vi "Command Editor Dialog 2.vi"(7 "Name(\"\" to use uuid)":string="Event CSM Tiny", 8 "Error in":errorcluster caption="Error in (no error)", 11 "CSM States":string="UI: Front Panel State >> Open -@ abc") -> (0 "Error out":errorcluster, 3 "Command out":string)   [LabVIEW 2017]
uses:
  user.lib/_NEVSTOP/Communicable State Machine(CSM)/_tool/_Support/def-message type.ctl
  user.lib/_NEVSTOP/Communicable State Machine(CSM)/_tool/_Support/def-Selection Type.ctl
  <vilib>/event_ctls.llb/eventvkey.ctl
  <vilib>/Utility/miscctls.llb/LVRowAndColumnUnsignedTypeDef.ctl
  user.lib/_NEVSTOP/Communicable State Machine(CSM)/AdvanceAPI/CSM - Keywords.vi
  user.lib/_NEVSTOP/Communicable State Machine(CSM)/_Support/Common/Trim Single line Text.vi
  user.lib/_NEVSTOP/Communicable State Machine(CSM)/AdvanceAPI/CSM - Break Down Multiple States String.vi
  user.lib/_NEVSTOP/Communicable State Machine(CSM)/AdvanceAPI/CSM - Compact Multiple States.vi
  user.lib/_NEVSTOP/Communicable State Machine(CSM)/Communicable State Machine.lvlib
  user.lib/_NEVSTOP/Communicable State Machine(CSM)/_tool/_Support/interfacebrowser.lvlib
  user.lib/_NEVSTOP/Communicable State Machine(CSM)/_tool/_Support/csm-tool-support.lvlib
  user.lib/_NEVSTOP/Communicable State Machine(CSM)/_csmHelper/API with lvcsm Support/CSM-Helper API with lvcsm Support.lvlib
  user.lib/_NEVSTOP/Communicable State Machine(CSM)/_csmHelper/CSM-Helper.lvclass
panel:
  out "current time":timestamp
  out "Selection":T2
  out "Msg Type":T3=enum."Message"
  in  "clear comments":bool
  in  "clear arguments":bool
  in  "->|":bool
  in  "->":bool
  in  "-@":bool
  in  "Interface-Filter":enum16{"API-Only", "UserDef States", "All"}(ring)=enum."UserDef States"
  in  "Candidates":i32(listbox)
  in  "MainTree":string(tree)
  in  "CSM-States":i32(listbox)
  in  "Comments":string
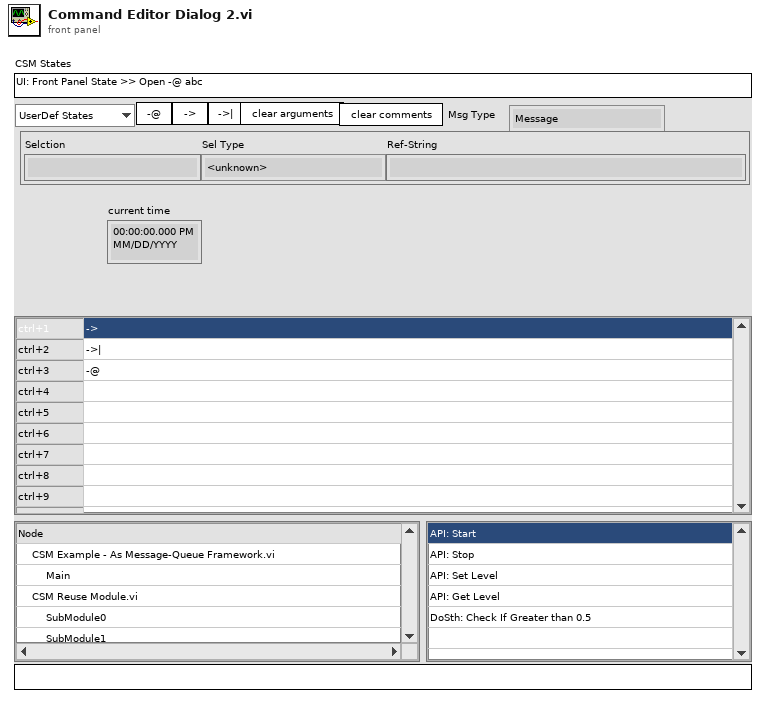
[diagram p1: front panel]
types:
  T1 = typedef "def-Selection Type.ctl" = enum16{"<unknown>", "State-StateOrSignal", "State-ArgSymbol", "State-Arg", "Reg-Oper", "Reg-Symbol", "Msg-State", "Msg-Arg", "Msg-ArgSymbol", "Msg-Symbol", "Msg-Module", "Broadcast-Signal", "Broadcast-ArgSymbol", "Broadcast-Arg", "Broadcast-Symbol", "Broadcast-Oper", "Comment-Symbol", "Comment-Content"}
  T2 = cluster{"Selction":string, "Sel Type":T1, "Ref-String":string}
  T3 = typedef "def-message type.ctl" = enum16{"State", "Message", "Broadcast", "Registration"}
  T4 = enum32{"Invalid", "Standard", "Closed", "Hidden", "Minimized", "Maximized"}
  T5 = enum32{"invalid app kind", "Development System", "Run Time System", "Student Edition", "Embedded LabVIEW", "Evaluation", "Custom"}
  T6 = typedef "LVRowAndColumnUnsignedTypeDef.ctl" = cluster{"Row":u32, "Column":u32}
  T7 = cluster{"Opton:All-CSM-VIs":bool, "Option:Online Only":bool}
  T8 = typedef "Communicable State Machine.lvlib/_CSM_Response Source Message.ctl" = cluster{"‘State":string, "’Arguments":string, "’Error":errorcluster}
  T9 = cluster{"Core":cluster{"Current VI Reference":refnum<vi>, "Close Panel on Exit?":bool}, "CSM States":string, "Selection":cluster{"end":i32, "start":i32}, "Msg Type":T3, "Selection":cluster{"Selction":string, "Sel Type":T1, "Ref-String":string}}
  T10 = typedef "LVPoint32TypeDef.ctl" = cluster{"Horizontal":i32, "Vertical":i32}
  T11 = typedef "eventvkey.ctl" = enum16{"ASCII", "Enter", "Return", "Shift", "Ctrl", "Alt", "Cmd", "Opt", "Caps", "NumLock", "Clear", "Break", "Up", "Down", "Left", "Right", "Insert", "Delete", "Home", "End", "PageUp", "PageDown", "Escape", "Help", "Pause", "ScrollLock", "F1", "F2", "F3", "F4", "F5", "F6", "F7", "F8", "F9", "F10", "F11", "F12", "F13", "F14", "F15", "F16", "F17", "F18", "F19", "F20", "F21", "F22", "F23", "F24", "Play", "VolumeUp", "VolumeDown", "Mute", "Two Byte Char"}
  T12 = cluster{"Shift":bool, "Ctrl":bool, "Alt":bool, "Cmd":bool, "Opt":bool}
  T13 = cluster{"Current VI Reference":refnum<vi>, "Close Panel on Exit?":bool}
  T14 = typedef "LVSelectionTypeDef.ctl" = cluster{"Selection Start":u32, "Selection End":u32}
  T15 = cluster{"single-line text":string, "single-line text":string}
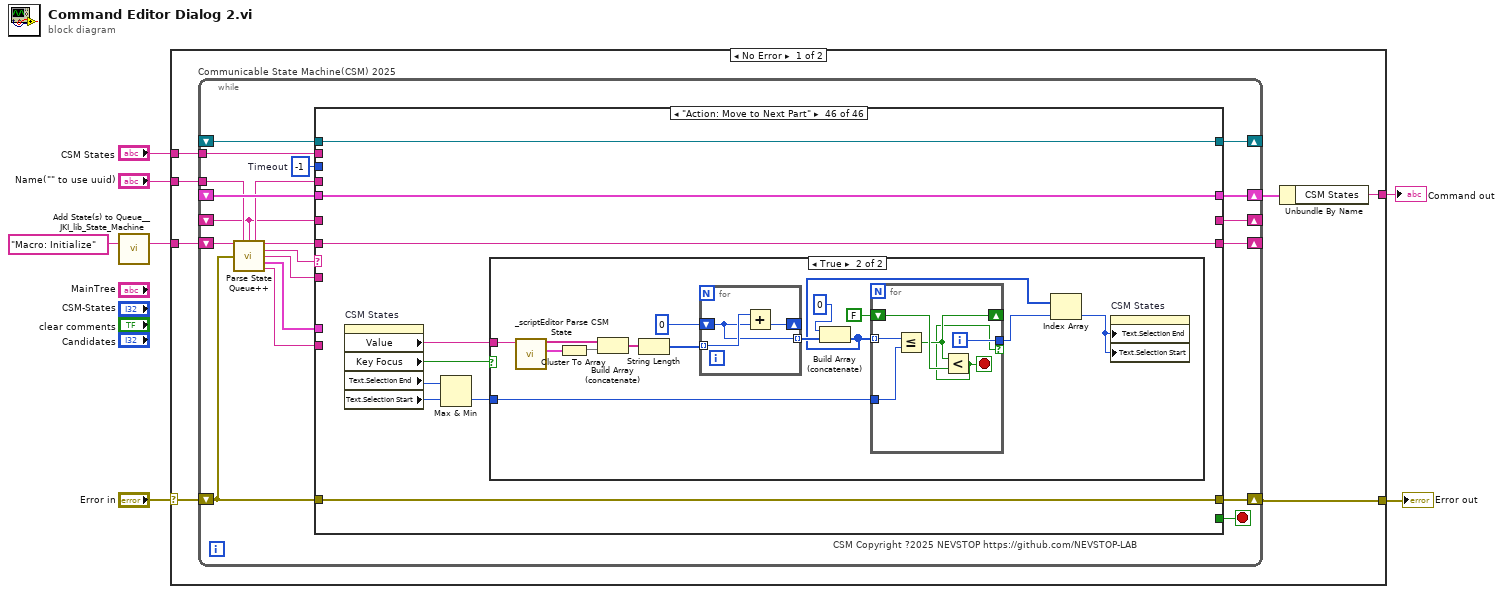
[diagram p0: block diagram]
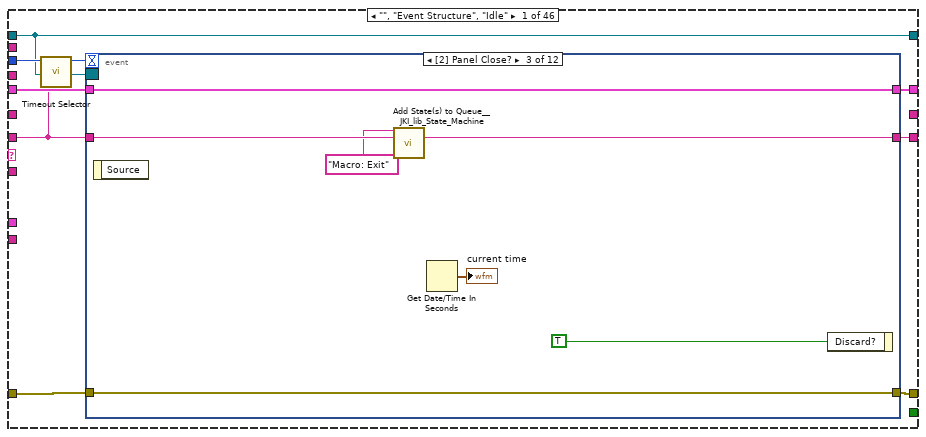
[diagram p2: hidden frame]
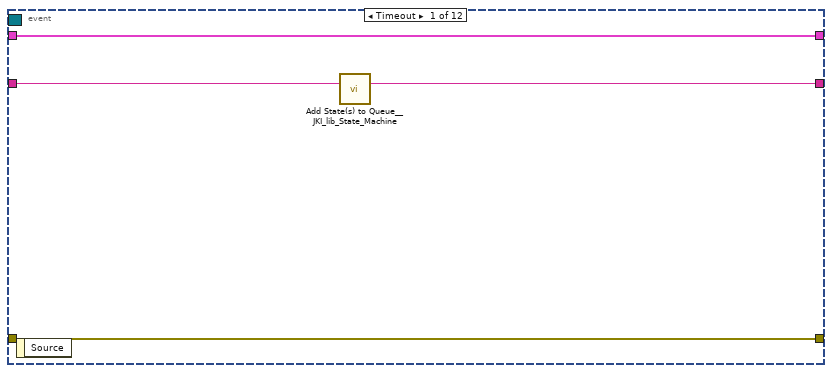
[diagram p3: hidden frame]
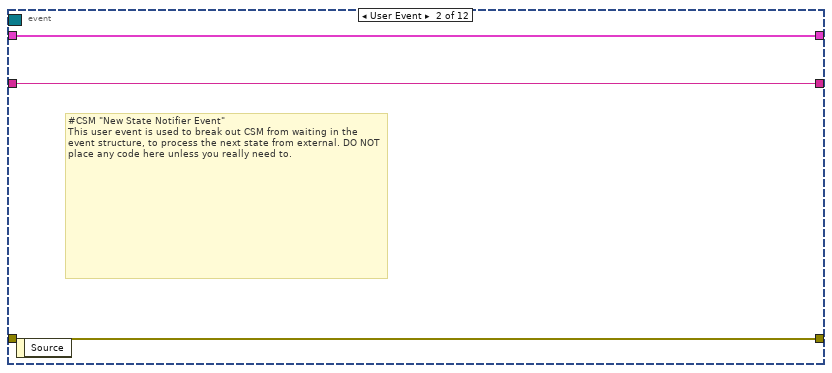
[diagram p4: hidden frame]
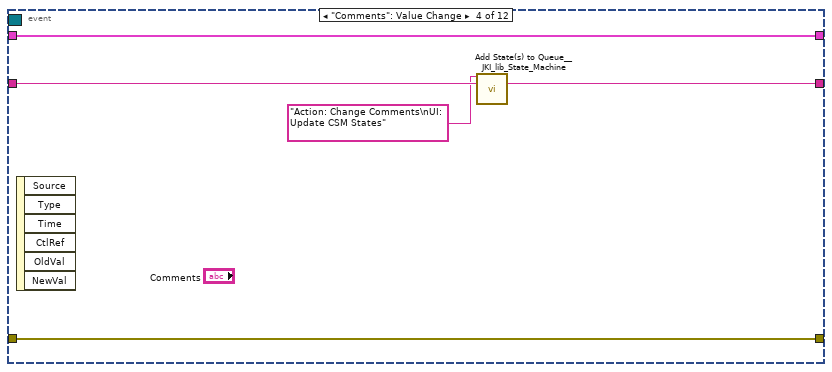
[diagram p5: hidden frame]
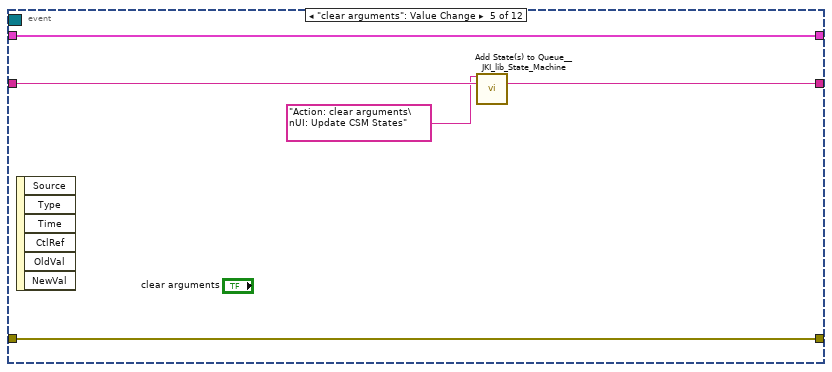
[diagram p6: hidden frame]
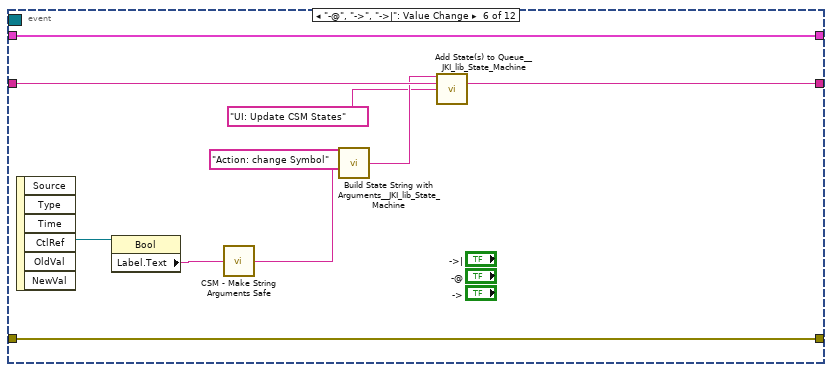
[diagram p7: hidden frame]
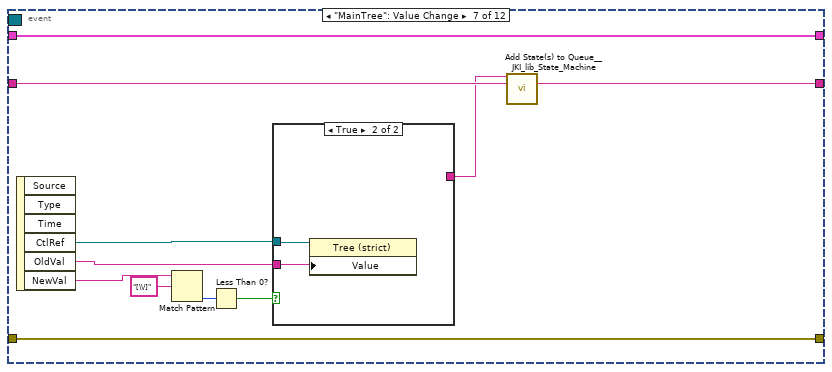
[diagram p8: hidden frame]
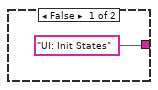
[diagram p9: hidden frame]
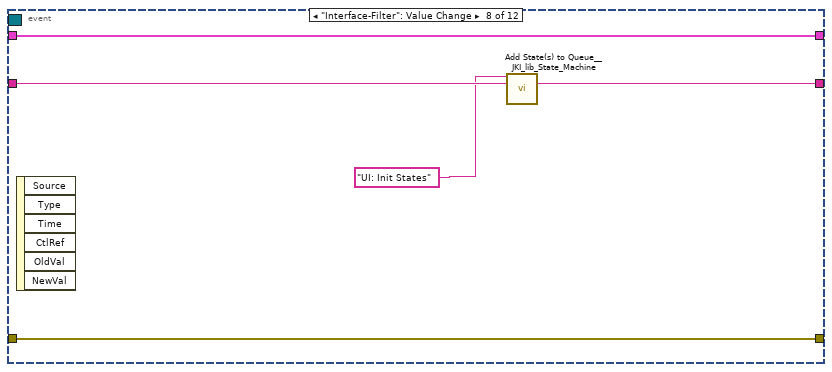
[diagram p10: hidden frame]
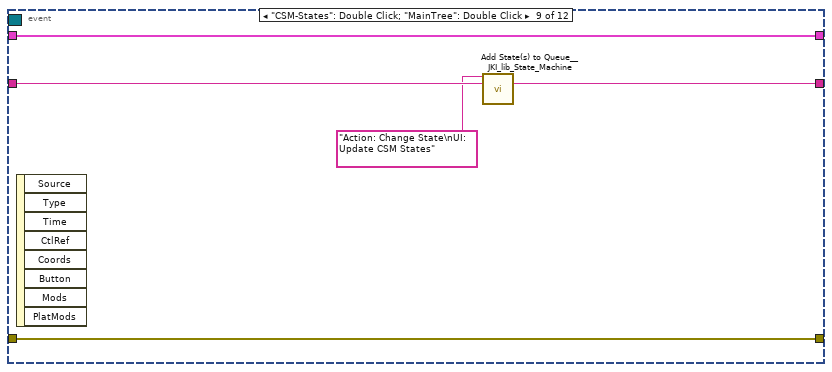
[diagram p11: hidden frame]
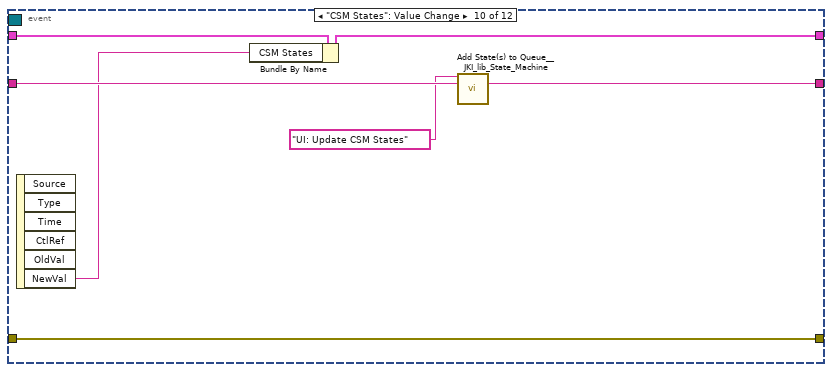
[diagram p12: hidden frame]
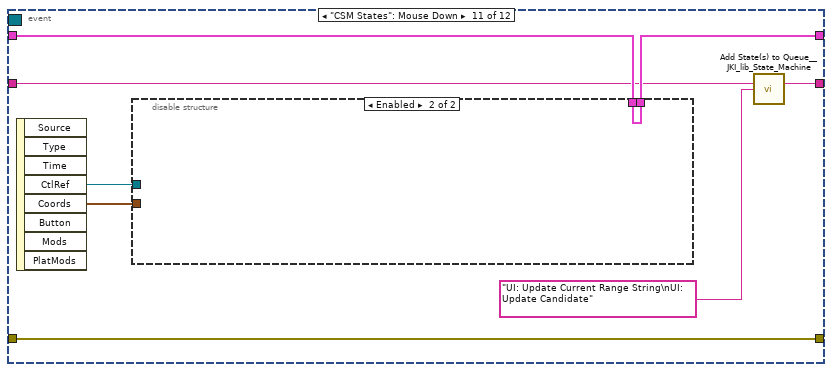
[diagram p13: hidden frame]
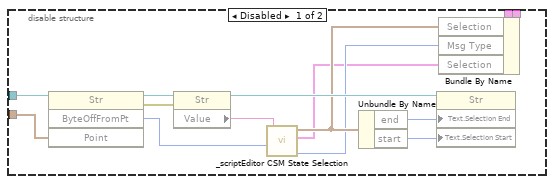
[diagram p14: hidden frame]
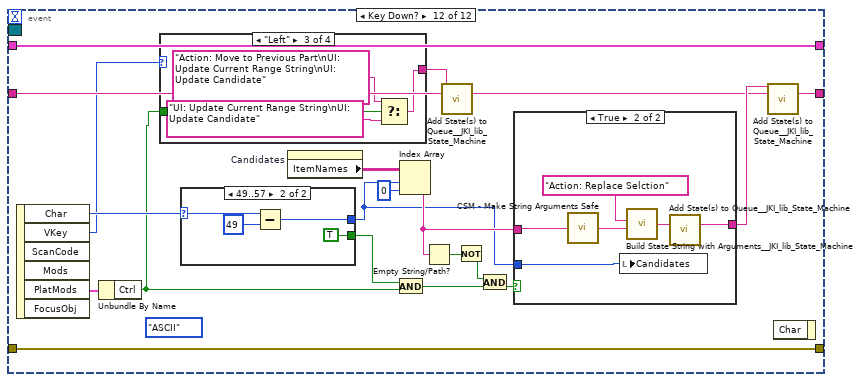
[diagram p15: hidden frame]
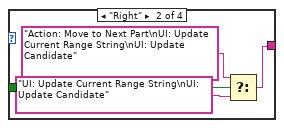
[diagram p17: hidden frame]
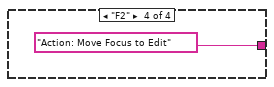
[diagram p18: hidden frame]
diagram:
  n1 = call <vilib>:"Add State(s) to Queue__JKI_lib_State_Machine.vi"("State(s) in (\"\")"="Macro: Initialize" ("Init State(\"Macro: Initialize\")")) -> ("States Out"=w7:string)  [unwired: 14 in]
  n2 = case shown="No Error" "Error in" {
    selector: "Error in" -> [w11 w791]
    tunnel: w7 -> [w14 _]
    tunnel: "Name(\"\" to use uuid)" -> [w13 _]
    tunnel: [w12 w791] -> w4
    tunnel: [w9 w790] -> w1
    tunnel: "CSM States" -> [w8 w790]
    frame No Error {
      n3 = while "Communicable State Machine(CSM) 2025" {
        shift-right: [w29] -> w10
        shift-left: _ -> [w28]
        shift-right: [w32] -> w12
        shift-left: w11 -> [w26]
        shift-right: [w31] -> _
        shift-left: w14 -> [w33]
        tunnel: w13 -> [w22]
        shift-right: [w25] -> _
        shift-left: _ -> [w16]
        shift-right: [w24] -> _
        shift-left: _ -> [w23]
        tunnel: w8 -> [w15]
        stop <- w30 stop-if-true
        w27 = -1  # Timeout
        # "CSM Copyright ?2025 NEVSTOP https://github.com/NEVSTOP-LAB"
        n4 = call "Parse State Queue++.vi"("State Queue"=w33, "Name(\"\" to use uuid)"=w22, "Response Arguments"=w16, "Previous Error"=w26) -> ("Name Used"=w17:string, "Remaining States"=w34:string, "Current State"=w21:string, "Arguments"=w20:string, ">> Response Source Message >>"=w19:T8, ">> Source CSM >>"=w18:string)  [unwired: 6 in]
        n5 = case shown="\"Action: Move to Next Part\"" w21 {
          selector: w21 -> [_ _ _ w182 _ _ _ _ _ _ _ _ _ _ _ _ _ _ _ _ _ _ _ _ _ _ _ _ _ _ _ _ _ _ _ _ _ _ _ _ _ _ _ _ _ _]
          tunnel: w34 -> [w35 w173 w179 w187 w194 w200 w223 w229 w236 w245 w258 w273 w279 w284 w294 w301 w306 w313 w317 w323 w331 w346 w367 w384 w402 w418 w491 w503 w507 w511 w523 w540 w546 w558 w561 w564 w576 w585 w605 w640 w668 w695 w700 w709 w732 w765]
          tunnel: w20 -> [_ _ _ _ _ w199 w218 w228 w235 w244 _ _ _ _ _ _ _ _ _ _ _ _ _ _ w397 w412 _ _ _ _ _ _ _ _ _ w566 _ _ w595 _ _ w688 _ _ _ _]
          tunnel: w28 -> [w42 w172 w176 w185 w193 w204 w224 w231 w238 w247 w257 w266 w277 w281 _ w296 w303 w312 w316 w320 w327 w345 w366 w387 w400 w414 w489 w497 w506 w510 w521 w537 w543 w555 w560 w570 w573 w583 w603 w638 w666 w692 w699 w708 w731 w764]
          tunnel: [w41 w174 w177 w180 w195 errorcluster {"status"=FALSE, "code"=0, "source"=""} ("error out") w219 w226 w233 w250 w259 w270 w276 w282 w291 w297 w304 w307 w315 w321 w329 w347 w368 w395 w398 w415 w492 w504 w508 w512 w524 w538 w544 w556 w562 w571 w574 w586 w606 w641 w669 w696 w701 w710 w733 w766] -> w32
          tunnel: w26 -> [w40 w174 w177 w188 w195 w201 w225 w227 w234 _ w259 w270 w276 w282 w291 w298 w304 _ w318 w321 w329 w347 w368 w395 w399 w416 w492 w504 w508 w512 w524 w538 w544 w556 w562 w571 w574 w586 w606 w641 w669 w696 w701 w710 w733 w766]
          tunnel: [w43 w173 w178 w186 w194 w196 w222 w232 w239 w246 w258 w272 w278 w283 w293 w300 w305 w313 w317 w322 w330 w346 w367 w385 w401 w417 w491 w503 w507 w511 w523 w539 w545 w557 w561 w565 w575 w585 w605 w640 w668 w695 w700 w709 w732 w765] -> w31
          tunnel: [_ _ _ _ _ _ TRUE _ _ _ _ _ TRUE _ _ _ _ _ _ _ _ _ _ _ _ _ _ _ _ _ _ _ _ _ _ _ _ _ _ _ _ _ _ _ _ _] -> w30
          tunnel: [w39 w172 w176 w185 w193 w204 w224 w231 w238 w248 w257 w271 w277 w281 w292 w296 w303 w312 w316 w320 w327 w345 w366 w387 w400 w414 w489 w496 w506 w510 w521 w537 w543 w555 w560 w568 w573 w579 w600 w635 w663 w693 w699 w708 w731 w764] -> w29
          tunnel: w27 -> [w38 _ _ _ _ _ _ _ _ _ _ _ _ _ _ _ _ _ _ _ _ _ _ _ _ _ _ _ _ _ _ _ _ _ _ _ _ _ _ _ _ _ _ _ _ _]
          tunnel: w18 -> [_ _ _ _ _ _ _ _ _ w242 _ _ _ _ _ _ _ _ _ _ _ _ _ _ _ _ _ _ _ _ _ _ _ _ _ _ _ _ _ _ _ _ _ _ _ _]
          tunnel: w19 -> [_ _ _ _ _ _ _ _ _ w249 _ _ _ _ _ _ _ _ _ _ _ _ _ _ _ _ _ _ _ _ _ _ _ _ _ _ _ _ _ _ _ _ _ _ _ _]
          tunnel: [_ _ _ "" w189 _ _ _ _ _ _ _ _ _ _ _ _ _ _ _ _ _ _ _ _ _ _ _ _ _ _ _ _ _ _ _ _ _ _ _ _ _ _ _ _ _] -> w25
          tunnel: [w37 w171 w175 w183 w192 w203 w220 w230 w237 w251 w256 w260 w274 w280 w289 w295 w302 w311 w314 w319 w328 w344 w365 w394 w396 w411 w490 w502 w505 w509 w522 w536 w541 w548 w559 w569 w572 w584 w604 w639 w667 w694 w698 w707 w730 w763] -> w24
          tunnel: w23 -> [w37 w171 w175 w183 w192 w203 w220 w230 w237 w251 w256 w260 w274 w280 w289 w295 w302 _ w314 w319 w328 w344 w365 w394 w396 w411 w490 w502 w505 w509 w522 w536 w541 w548 w559 w569 w572 w584 w604 w639 w667 w694 w698 w707 w730 w763]
          tunnel: w17 -> [_ _ _ w181 _ _ w217 _ _ _ _ _ _ _ _ _ _ w310 _ _ _ _ _ _ _ _ _ _ _ _ _ _ _ _ _ _ _ _ _ _ _ _ _ _ _ _]
          tunnel: w16 -> [_ _ _ _ _ _ _ _ _ _ _ _ _ _ _ _ _ _ _ _ _ _ _ _ _ _ _ _ _ _ _ _ _ _ _ _ _ _ _ _ _ _ _ _ _ _]
          tunnel: w15 -> [_ _ _ _ _ _ _ _ _ _ _ _ _ _ w288 _ _ _ _ _ _ _ _ _ _ _ _ _ _ _ _ _ _ _ _ _ _ _ _ _ _ _ _ _ _ _]
          frame "", "Event Structure", "Idle" {
            n6 = call "Timeout Selector.vi"("Remaining States"=w35, "Timeout Expected"=w38) -> ("Timeout"=w36:i32)  [unwired: 5 in]
            n7 = event shown="[2] Panel Close?" {
              selector: w37 -> [_ _ _ _ _ _ _ _ _ _ _ _]
              dyn-events: _ -> [_ _ _ _ _ _ _ _ _ _ _ _]
              timeout: w36 -> [_ _ _ _ _ _ _ _ _ _ _ _]
              tunnel: w35 -> [w47 w49 w57 w59 w64 w74 w79 w93 w98 w105 w110 w136]
              tunnel: [w46 w49 w56 w60 w65 w75 w80 w94 w99 w106 w111 w147] -> w43
              tunnel: w42 -> [w44 w50 w54 w61 w66 w76 w87 w95 w100 w107 w115 w150]
              tunnel: [w45 w48 w55 w62 w67 w77 w88 w96 w101 w108 w116 w151] -> w41
              tunnel: w40 -> [w45 w48 w55 w62 w67 w77 w88 w96 w101 w108 w116 w151]
              tunnel: [w44 w50 w54 w61 w66 w76 w87 w95 w100 w103 w112 w150] -> w39
              event Timeout {
                n8 = event-data() -> ()  [unwired: 1 in, 1 out]
                n9 = call <vilib>:"Add State(s) to Queue__JKI_lib_State_Machine.vi"("State(s) in (\"\")"=w47) -> ("States Out"=w46:string)  [unwired: 14 in]
              }
              event User Event {
                # "#CSM \"New State Notifier Event\"\nThis user event is used to break out CSM from waiting in the event structure, to process the next state from external. DO NOT place any code here unless you really need to."
                n10 = event-data() -> ()  [unwired: 1 in, 1 out]
              }
              event Panel Close? {
                n11 = event-data() -> ()  [unwired: 1 in, 1 out]
                n12 = call <vilib>:"Add State(s) to Queue__JKI_lib_State_Machine.vi"("State(s) in Front (\"\")"="Macro: Exit", "State(s) in (\"\")"=w57) -> ("States Out"=w56:string)  [unwired: 13 in]
                n13 = Get Date/Time In Seconds() -> (seconds since 1Jan1904=→"current time":timestamp)
                n14 = event-data("Discard?"=TRUE) -> ()  [unwired: 1 in, 1 out]
              }
              event "Comments": Value Change {
                n15 = event-data() -> ()  [unwired: 1 in, 6 out]
                n16 = call <vilib>:"Add State(s) to Queue__JKI_lib_State_Machine.vi"("State(s) in Front (\"\")"="Action: Change Comments\nUI: Update CSM States" ("State(s) in Front (\"\")"), "State(s) in (\"\")"=w59) -> ("States Out"=w60:string)  [unwired: 13 in]
              }
              event "clear arguments": Value Change {
                n17 = event-data() -> ()  [unwired: 1 in, 6 out]
                n18 = call <vilib>:"Add State(s) to Queue__JKI_lib_State_Machine.vi"("State(s) in Front (\"\")"="Action: clear arguments\nUI: Update CSM States" ("State(s) in Front (\"\")"), "State(s) in (\"\")"=w64) -> ("States Out"=w65:string)  [unwired: 13 in]
              }
              event "-@", "->", "->|": Value Change {
                n19 = event-data() -> ("CtlRef"=w71:refnum<vi>)  [unwired: 1 in, 5 out]
                n20 = property class="Bool"(reference=w71) -> ("Label.Text"=w70:string)  [unwired: 1 in, 2 out]
                n21 = call "CSM - Make String Arguments Safe.vi"("Argurment String"=w70) -> ("Safe Argurment String"=w69:string)  [unwired: 8 in]
                n22 = call <vilib>:"Build State String with Arguments__JKI_lib_State_Machine.vi"("Arguments (\"\")"=w69, "State"="Action: change Symbol") -> ("State with Arguments"=w73:string)  [unwired: 4 in]
                n23 = call <vilib>:"Add State(s) to Queue__JKI_lib_State_Machine.vi"("State(s) in Front (\"\")"=w73, "State(s) in (\"\")"=w74, "State(s) at Back (\"\")"="UI: Update CSM States" ("State")) -> ("States Out"=w75:string)  [unwired: 12 in]
              }
              event "MainTree": Value Change {
                n24 = event-data() -> ("CtlRef"=w82:refnum<vi>, "OldVal"=w81:string, "NewVal"=w86:string)  [unwired: 1 in, 3 out]
                n25 = Match Pattern(string=w86, regular expression="[\\/]") -> (offset past match=w84:i32)  [unwired: 1 in, 3 out]
                n26 = Less Than 0?(x=w84) -> (x < 0?=w83:bool)
                n27 = case shown="True" w83 {
                  tunnel: w82 -> [_ w91]
                  tunnel: w81 -> [_ w90]
                  tunnel: ["UI: Init States" ("State(s) in Front (\"\")") _] -> w78
                  frame False {
                  }
                  frame True {
                    n28 = property class="Tree (strict)"(reference=w91, "Value"=w90) -> ()  [unwired: 1 in, 2 out]
                  }
                }
                n29 = call <vilib>:"Add State(s) to Queue__JKI_lib_State_Machine.vi"("State(s) in Front (\"\")"=w78, "State(s) in (\"\")"=w79) -> ("States Out"=w80:string)  [unwired: 13 in]
              }
              event "Interface-Filter": Value Change {
                n30 = event-data() -> ()  [unwired: 1 in, 6 out]
                n31 = call <vilib>:"Add State(s) to Queue__JKI_lib_State_Machine.vi"("State(s) in Front (\"\")"="UI: Init States" ("State(s) in Front (\"\")"), "State(s) in (\"\")"=w93) -> ("States Out"=w94:string)  [unwired: 13 in]
              }
              event "CSM-States", "MainTree": Double Click {
                n32 = event-data() -> ()  [unwired: 1 in, 8 out]
                n33 = call <vilib>:"Add State(s) to Queue__JKI_lib_State_Machine.vi"("State(s) in Front (\"\")"="Action: Change State\nUI: Update CSM States" ("State(s) in Front (\"\")"), "State(s) in (\"\")"=w98) -> ("States Out"=w99:string)  [unwired: 13 in]
              }
              event "CSM States": Value Change {
                n34 = event-data() -> ("NewVal"=w102:string)  [unwired: 1 in, 5 out]
                n35 = Bundle By Name(cluster=w107, "CSM States"=w102) -> (w103:T9)
                n36 = call <vilib>:"Add State(s) to Queue__JKI_lib_State_Machine.vi"("State(s) in Front (\"\")"="UI: Update CSM States" ("State(s) in Front (\"\")"), "State(s) in (\"\")"=w105) -> ("States Out"=w106:string)  [unwired: 13 in]
              }
              event "CSM States": Mouse Down {
                n37 = event-data() -> ("CtlRef"=w114:refnum<vi>, "Coords"=w113:T10)  [unwired: 1 in, 6 out]
                n38 = disable-structure shown="Enabled" {
                  disable-tunnel: w115 -> [w130 w131]
                  disable-tunnel: w114 -> [w129 _]
                  disable-tunnel: w113 -> [w128 _]
                  disable-tunnel: [w120 w131] -> w112
                  frame Disabled {
                    n39 = invoke class="Str" method="ByteOffFromPt"(reference=w129, "Point"=w128) -> (reference out=w127:refnum<vi>, error out=w126:errorcluster, "ByteOffFromPt"=w123:i32)  [unwired: 2 in, 1 out]
                    n40 = property class="Str"(reference=w127, error in=w126) -> (reference out=w125:refnum<vi>, "Value"=w124:string)  [unwired: 1 out]
                    n41 = call "_scriptEditor CSM State Selection.vi"("Pos"=w123, "single-line text"=w124) -> ("Msg Type"=w118:T3, "Selection"=w117:T2, "Selection 2"=w119:cluster{"end":i32, "start":i32})  [unwired: 7 in]
                    n42 = Unbundle By Name(w119) -> ("end"=w122:i32, "start"=w121:i32)
                    n43 = property class="Str"(reference=w125, "Text.Selection End"=w122, "Text.Selection Start"=w121) -> ()  [unwired: 1 in, 2 out]
                    n44 = Bundle By Name(cluster=w130, "Selection"=w119, "Msg Type"=w118, "Selection"=w117) -> (w120:T9)
                  }
                  frame Enabled {
                  }
                }
                n45 = call <vilib>:"Add State(s) to Queue__JKI_lib_State_Machine.vi"("State(s) in (\"\")"=w110, "State(s) at Back (\"\")"="UI: Update Current Range String\nUI: Update Candidate" ("State(s) at Back (\"\")")) -> ("States Out"=w111:string)  [unwired: 13 in]
              }
              event Key Down? {
                (unwired) eventvkey."ASCII" ("VKey")
                n46 = event-data() -> ("Char"=w138:i16, "VKey"=w134:T11, "PlatMods"=w149:T12)  [unwired: 1 in, 3 out]
                n47 = Unbundle By Name(w149) -> ("Ctrl"=w132:bool)
                n48 = case shown="\"Left\"" w134 {
                  tunnel: [_ w152 w156 "Action: Move Focus to Edit" ("State(s) in Front (\"\")")] -> w135
                  tunnel: w132 -> [_ w155 w159 _]
                  frame "ASCII", Default {
                  }
                  frame "Right" {
                    n49 = Select(t="Action: Move to Next Part\nUI: Update Current Range String\nUI: Update Candidate" ("State(s) in Front (\"\")"), s=w155, f="UI: Update Current Range String\nUI: Update Candidate" ("State(s) in Front (\"\")")) -> (s? t:f=w152:string)
                  }
                  frame "Left" {
                    n50 = Select(t="Action: Move to Previous Part\nUI: Update Current Range String\nUI: Update Candidate" ("State(s) in Front (\"\")"), s=w159, f="UI: Update Current Range String\nUI: Update Candidate" ("State(s) in Front (\"\")")) -> (s? t:f=w156:string)
                  }
                  frame "F2" {
                  }
                }
                n51 = case shown="49..57" w138 {
                  selector: w138 -> [_ w170]
                  tunnel: [_ w168] -> w133
                  tunnel: [_ TRUE] -> w148
                  frame 0, Default {
                  }
                  frame 49..57 {
                    n52 = Subtract(x=w170, y=i16 49) -> (x-y=w168:i16)
                  }
                }
                n53 = property on="Candidates" class="MCListbox (strict)"() -> ("ItemNames"=w145:string[][])  [unwired: 2 in, 2 out]
                n54 = And(x=w148, y=w132) -> (x .and. y?=w146:bool)
                n55 = Index Array(array=w145, index (row)=w133, index (col)=0 ("disabled index (col)")) -> (element=w141:string)
                n56 = Empty String/Path?(string/path=w141) -> (empty?=w143:bool)
                n57 = call <vilib>:"Add State(s) to Queue__JKI_lib_State_Machine.vi"("State(s) in Front (\"\")"=w135, "State(s) in (\"\")"=w136) -> ("States Out"=w137:string)  [unwired: 13 in]
                n58 = Not(x=w143) -> (.not. x?=w142:bool)
                n59 = And(x=w142, y=w146) -> (x .and. y?=w139:bool)
                n60 = case shown="True" w139 {
                  tunnel: w141 -> [_ w166]
                  tunnel: [_ w163] -> w140
                  tunnel: w133 -> [_ w161]
                  frame False {
                  }
                  frame True {
                    n61 = call "CSM - Make String Arguments Safe.vi"("Argurment String"=w166) -> ("Safe Argurment String"=w162:string)  [unwired: 8 in]
                    n62 = local write "Candidates"(w161) -> ()
                    n63 = call <vilib>:"Build State String with Arguments__JKI_lib_State_Machine.vi"("Arguments (\"\")"=w162, "State"="Action: Replace Selction") -> ("State with Arguments"=w164:string)  [unwired: 4 in]
                    n64 = call <vilib>:"Add State(s) to Queue__JKI_lib_State_Machine.vi"("State(s) in (\"\")"=w164) -> ("States Out"=w163:string)  [unwired: 14 in]
                  }
                }
                n65 = call <vilib>:"Add State(s) to Queue__JKI_lib_State_Machine.vi"("State(s) in Front (\"\")"=w140, "State(s) in (\"\")"=w137) -> ("States Out"=w147:string)  [unwired: 13 in]
                n66 = event-data() -> ()  [unwired: 2 in, 1 out]
              }
            }
          }
          frame "CSM Documentation" {
          }
          frame "---------- Core ----------" {
            # "#CSM \"Category Seperator\"\nDo not put any code in this frame."
            n67 = call <vilib>:"Add State(s) to Queue__JKI_lib_State_Machine.vi"("State(s) in (\"\")"=w179) -> ("States Out"=w178:string)  [unwired: 14 in]
          }
          frame Default {
            # "#CSM \"Default\"\nthis is used to capture unhandled states and typos"
            # "Handle mistyped state name (developer tool)"
            n68 = call "CSM Unhandled State Error.vi"("error in (no error)"=w188, "Current State"=w182, "CSM Name"=w181) -> ("error out"=w180:errorcluster)  [unwired: 8 in]
            n69 = call <vilib>:"Add State(s) to Queue__JKI_lib_State_Machine.vi"("State(s) in (\"\")"=w187) -> ("States Out"=w186:string)  [unwired: 14 in]
          }
          frame "VI Reference" {
            n70 = Unbundle By Name(w193) -> ("Core"=w191:T13)
            n71 = Unbundle By Name(w191) -> ("Current VI Reference"=w190:refnum<vi>)
            n72 = call "CSM - Convert Data to HexStr.vi"("Variant"=w190) -> ("HEX String (0-9,A-F)"=w189:string)  [unwired: 8 in]
          }
          frame "Error Handler" {
            # "#CSM Disable this error dialog if you need"
            # "#CSM \"Error Handler\"\nYou can also output any states to clean-up after errors occur"
            # "Clear error"
            n73 = case shown="Error" w201 {
              selector: w201 -> [_ w211]
              tunnel: [w210 w213] -> w197
              tunnel: w200 -> [w210 w212]
              tunnel: w199 -> [w209 _]
              tunnel: [w208 w211] -> w202
              frame No Error {
                n74 = call "CSM - Convert Argument to Error.vi"("Argument"=w209) -> ("error"=w208:errorcluster)  [unwired: 4 in]
                n75 = flat-sequence {
                  frame #0 {
                    # "#CSM External Error Handler Case\nUsually, it's because This CSM register others' \"Error Occurred\" status with \"Error Handler\". If other CSM have any error, the error will be passed here for central handling."
                  }
                }
              }
              frame Error {
                # "#CSM Internal Error Handler Case \nIf any error Occurred, \"Error Occurred\" \nstatus update will be broadcasted to system.\nParameter is Error Cluster."
                n76 = call "CSM - Convert Error to Argument.vi"("error"=w211) -> ("Argument"=w215:string)  [unwired: 4 in]
                n77 = call <vilib>:"Build State String with Arguments__JKI_lib_State_Machine.vi"("Arguments (\"\")"=w215, "State"="Error Occurred" ("Status with Arguments")) -> ("State with Arguments"=w214:string)  [unwired: 4 in]
                n78 = call "CSM - Broadcast Status Change.vi"("Status with Arguments"=w214, "State Queue"=w212) -> ("Remaining States"=w213:string)  [unwired: 13 in]
              }
            }
            n79 = disable-structure shown="Enabled" {
              disable-tunnel: w202 -> [w206 w207]
              frame Enabled {
                n80 = call <vilib>:"General Error Handler.vi"("error in (no error)"=w206) -> ()  [unwired: 10 in, 5 out]
              }
              frame Disabled {
                n81 = call <vilib>:"Clear Errors.vi"("error in (no error)"=w207) -> ()  [unwired: 5 in, 2 out]
              }
            }
            n82 = call <vilib>:"Add State(s) to Queue__JKI_lib_State_Machine.vi"("State(s) in Front (\"\")"="// Post Error States", "State(s) in (\"\")"=w197) -> ("States Out"=w196:string)  [unwired: 13 in]
          }
          frame "Critical Error" {
            # "#CSM Stop in Critical Error\nWhen Critical Error occurs, Stop the loop immediately. Do NOT change this unless you fully understand the impact."
            # "#CSM \"Critical Error\"\nWhen any un-recoverable error occurs, CSM goes into this case."
            n83 = call "CSM Critical Error.vi"("error in (no error)"=w225, "Arugments(as Reason)"=w218, "CSM Name"=w217) -> ("error out"=w219:errorcluster)  [unwired: 8 in]
            n84 = call <vilib>:"Add State(s) to Queue__JKI_lib_State_Machine.vi"("State(s) in (\"\")"=w223) -> ("States Out"=w222:string)  [unwired: 14 in]
          }
          frame "Target Error" {
            # "#CSM \"Target Error\"\nWhen This CSM try to communicate with an un-existed CSM, This CSM goes into this case."
            n85 = call "CSM Target Error.vi"("error in (no error)"=w227, "Arguments(as CSM Name)"=w228) -> ("error out"=w226:errorcluster)  [unwired: 9 in]
            n86 = call <vilib>:"Add State(s) to Queue__JKI_lib_State_Machine.vi"("State(s) in (\"\")"=w229) -> ("States Out"=w232:string)  [unwired: 14 in]
          }
          frame "Target Timeout Error" {
            # "#CSM \"Target Timeout Error\"\nWhen This CSM could not get the sync-call response in time, This CSM goes into this case."
            n87 = call "CSM Target Timeout Error.vi"("error in (no error)"=w234, "Arguments(as CSM Name)"=w235) -> ("error out"=w233:errorcluster)  [unwired: 9 in]
            n88 = call <vilib>:"Add State(s) to Queue__JKI_lib_State_Machine.vi"("State(s) in (\"\")"=w236) -> ("States Out"=w239:string)  [unwired: 14 in]
          }
          frame "Async Response", "Response" {
            n89 = Unbundle(w249) -> ("‘State"=w243:string, "’Arguments"=w241:string, "’Error"=w240:errorcluster)
            n90 = case shown="Default" w243 {
              tunnel: [w255] -> w250
              tunnel: w240 -> [w255]
              tunnel: [w254] -> w248
              tunnel: w247 -> [w254]
              tunnel: [w252] -> w246
              tunnel: w245 -> [w253]
              tunnel: w244 -> [_]
              tunnel: w242 -> [_]
              tunnel: w241 -> [_]
              frame Default {
                # "#CSM Response Comments\nAfter Message is executed, CSM goes to this state for receive the response.\n    For Async Message(->), \"Async Response\" is used. This CSM will goes to \"Async Message Posted\" immediately and receive the \"Async Response\" after the callee finishes the message.\n    For Sync Message(@),  This CSM will wait until the message is done and immediately goes to \"Response\""
                # "#CSM \"Async Response\"\nHandle Async-call Response (\"Async Response\" for ->)"
                # "#CSM \"Response\"\nHandle Sync-call Response (\"Response\" for -@)"
                n91 = call <vilib>:"Add State(s) to Queue__JKI_lib_State_Machine.vi"("State(s) in (\"\")"=w253) -> ("States Out"=w252:string)  [unwired: 14 in]
              }
            }
          }
          frame "Async Message Posted" {
            # "#CSM \"Async Message Posted\"\nAfter Async Message is posted (-> or ->| ), CSM goes to this state for post-action.\nYou can use Argument - State to tell which Async Message is called."
          }
          frame "Initialize Core Data" {
            # "#CSM \"Initialize Core Data\"\nThis is used to determine panel behavior on exit"
            # "originally closed?"
            # "exe?"
            # "If panel starts closed or is an EXE, then close it when we exit"
            n92 = property class="VI"() -> ("FP.State"=w263:T4)  [unwired: 2 in, 2 out]
            n93 = property class="App"() -> ("App.Kind"=w269:T5)  [unwired: 2 in, 2 out]
            n94 = control-ref of="Current VI Reference"() -> (w264:refnum<vi>)
            n95 = Equal?(x=w263, y=T4."Closed" ("Front Panel Window:State")) -> (x = y?=w261:bool)
            n96 = Equal?(x=w269, y=T5."Run Time System" ("Application:Kind")) -> (x = y?=w267:bool)
            n97 = Or(x=w261, y=w267) -> (x .or. y?=w265:bool)
            n98 = Bundle By Name(cluster=w266, "Core.Current VI Reference"=w264, "Core.Close Panel on Exit?"=w265) -> (w271:T9)
            n99 = call <vilib>:"Add State(s) to Queue__JKI_lib_State_Machine.vi"("State(s) in (\"\")"=w273) -> ("States Out"=w272:string)  [unwired: 14 in]
          }
          frame "Exit" {
            # "#CSM \"Exit\"\nCase for exiting the loop. No errors that occur here will be handled."
            n100 = call <vilib>:"Add State(s) to Queue__JKI_lib_State_Machine.vi"("State(s) in (\"\")"=w279) -> ("States Out"=w278:string)  [unwired: 14 in]
          }
          frame "---------- Data ----------" {
            # "#CSM \"Category Seperator\"\nDo not put any code in this frame."
            n101 = call <vilib>:"Add State(s) to Queue__JKI_lib_State_Machine.vi"("State(s) in (\"\")"=w284) -> ("States Out"=w283:string)  [unwired: 14 in]
          }
          frame "Data: Initialize" {
            w285 = T2 {"Selction"="<register>", "Sel Type"=enum."Reg-Oper", "Ref-String"=""}  # Selection
            w287 = cluster{"end":i32, "start":i32} {"end"=0, "start"=0}  # Selection
            w286 = def-message_type."Registration"  # Msg Type
            w290 = T13 {"Current VI Reference"=refnum, "Close Panel on Exit?"=FALSE}  # Core
            n102 = call <vilib>:"Add State(s) to Queue__JKI_lib_State_Machine.vi"("State(s) in (\"\")"=w294) -> ("States Out"=w293:string)  [unwired: 14 in]
            n103 = Bundle("Core"=w290, "CSM States"=w288, "Selection"=w287, "Msg Type"=w286, "Selection"=w285) -> (w292:T9)  [unwired: 1 in]
          }
          frame "Data: Cleanup" {
            # "Cleanup any data and references, here.\n(this is called automatically, by the Macro: Exit)"
            n104 = Unbundle By Name(w296) -> ("Core.Current VI Reference"=w299:refnum<vi>)
            n105 = Close Reference(reference=w299, error in (no error)=w298) -> (error out=w297:errorcluster)
            n106 = call <vilib>:"Add State(s) to Queue__JKI_lib_State_Machine.vi"("State(s) in (\"\")"=w301) -> ("States Out"=w300:string)  [unwired: 14 in]
          }
          frame "---------- Events ----------" {
            # "#CSM \"Category Seperator\"\nDo not put any code in this frame."
            n107 = call <vilib>:"Add State(s) to Queue__JKI_lib_State_Machine.vi"("State(s) in (\"\")"=w306) -> ("States Out"=w305:string)  [unwired: 14 in]
          }
          frame "Events: Register" {
            # "#CSM \"Events: Register\"\nRegister user event. New Message Event is registered to break CSM waiting in event structure by default."
            # "#CSM Register New Message Event\nRegister message event to break Waiting in Event structure."
            n108 = call "CSM - Get New State Notifier Event.vi"("Name(\"\" to use uuid) in"=w310) -> ("Error out"=w308:errorcluster, "New State Notifier Event"=w309:refnum<user-event>)  [unwired: 9 in]
            n109 = register-events(error in=w308, w309) -> (reference out=w311:refnum<event-registration>, error out=w307:errorcluster)  [unwired: 1 in]
          }
          frame "Events: Unregister" {
            # "#CSM \"Events: Unregister\"\nUnregister user event."
            n110 = Unregister For Events(event registration refnum=w314, error in=w318) -> (error out=w315:errorcluster)
          }
          frame "---------- UI ----------" {
            # "#CSM \"Category Seperator\"\nDo not put any code in this frame."
            n111 = call <vilib>:"Add State(s) to Queue__JKI_lib_State_Machine.vi"("State(s) in (\"\")"=w323) -> ("States Out"=w322:string)  [unwired: 14 in]
          }
          frame "UI: Initialize" {
            n112 = for {
              N: 9 -> [_]
              tunnel: [w333] -> w325 mode=indexing
              i -> [w335]
              n113 = Increment(x=w335) -> (x+1=w332:i32)
              n114 = Format Into String(format string="ctrl+%d", w332) -> (resulting string=w333:string)  [unwired: 2 in, 1 out]
            }
            n115 = property on="Candidates" class="MCListbox (strict)"("RowHdrs[]"=w325, "TopLeft"=T6 {"Row"=0, "Column"=0} ("Top Left Visible Cell")) -> ()  [unwired: 2 in, 2 out]
            n116 = call <vilib>:"Add State(s) to Queue__JKI_lib_State_Machine.vi"("State(s) in (\"\")"=w331) -> ("States Out"=w330:string)  [unwired: 14 in]
          }
          frame "UI: Init MainTree" {
            n117 = control-ref of="MainTree"() -> (w337:refnum<vi>)
            n118 = call "_interfacebrowser build tree table in CSM-VI mode.vi"("Option"=T7 {"Opton:All-CSM-VIs"=FALSE, "Option:Online Only"=FALSE}) -> ("Type"=w343:string[], "Tree Table"=w342:string[][])  [unwired: 8 in, 1 out]
            n119 = call "Populate Tree with Delimited Strings_csm.vi"("Default Symbol"=0, "Delimiter"="/", "Items (Delimited)"=w342, "Tree Control"=w337) -> ("error out"=w340:errorcluster, "Tree Control Dup"=w341:refnum<vi>)  [unwired: 5 in, 1 out]
            n120 = property class="Tree"(reference=w341, error in=w340, "RowHdrs[]"=w343) -> ()  [unwired: 2 out]
          }
          frame "UI: Init States" {
            n121 = control-ref of="MainTree"() -> (w362:refnum<vi>)
            n122 = property class="Tree (strict)"(reference=w362) -> ("Value"=w363:string)  [unwired: 1 in, 2 out]
            n123 = Build Array(w363) -> (w353:string[])
            n124 = for {
              tunnel: [w381] -> w355 mode=indexing
              tunnel: w353 -> [w379] mode=indexing
              n125 = Match Pattern(string=w379, regular expression="/") -> (before substring=w378:string)  [unwired: 1 in, 3 out]
              n126 = call "Read CSM States By CSM-VI.vi"("CSM VI"=w378) -> ("Array"=w382:string[])  [unwired: 9 in, 1 out]
              n127 = Bundle("Array"=w382) -> (w381:cluster{"Array":string[]})  [unwired: 1 in]
            }
            n128 = Delete From Array(array=w355, index=0) -> (deleted portion=w357:cluster{"Array":string[]}, array with subset deleted=w356:cluster{"Array":string[]}[])  [unwired: 1 in]
            n129 = Unbundle(w357) -> ("Array"=w358:string[])
            n130 = for {
              tunnel: w356 -> [w374] mode=indexing
              shift-right: [w369] -> w359
              shift-left: w358 -> [w373]
              n131 = Unbundle(w374) -> ("Array"=w372:string[])
              n132 = Build Array (concatenate)(w373, w372) -> (w370:string[])
              n133 = call "_Remove Duplicates Strings.vi"("Input Array"=w370) -> ("indices of removed elements"=w371:i32[])  [unwired: 1 out]
              n134 = for {
                tunnel: w371 -> [w376] mode=indexing
                tunnel: w370 -> [w377]
                tunnel: [w375] -> w369 mode=indexing
                n135 = Index Array(array=w377, index=w376) -> (element=w375:string)
              }
            }
            n136 = control-ref of="CSM-States"() -> (w364:refnum<vi>)
            n137 = call "filter CSM States.vi"("Interface-Filter"="Interface-Filter", "Array"=w359) -> ("filtered array"=w360:string[])  [unwired: 9 in]
            n138 = property on="Property Node" class="LstBox (strict)"(reference=w364, "Item Names"=w360) -> (reference out=w352:refnum<vi>, "Value"=w350:i32)  [unwired: 1 in, 1 out]
            n139 = Less Than 0?(x=w350) -> (x < 0?=w351:bool)
            n140 = Select(t=0, s=w351, f=w350) -> (s? t:f=w348:i32)
            n141 = property on="Property Node" class="LstBox (strict)"(reference=w352, "Value"=w348) -> ()  [unwired: 1 in, 2 out]
          }
          frame "UI: Refresh Inputs" {
            n142 = Unbundle By Name(w387) -> ("CSM States"=w386:string)
            n143 = call "Remove Comments from Line.vi"("single-line text"=w386) -> ("single-line text without comments"=w392:string)  [unwired: 2 in]
            n144 = call "Splite Single-line Message.vi"("single-line text"=w392) -> ()  [unwired: 6 in, 4 out]
            n145 = String Length(string=w392) -> (length=w393:i32)
            n146 = String Subset(string=w386, offset (0)=w393) -> (substring=w390:string)  [unwired: 1 in]
            n147 = call "Trim Both Whitespace.vi"("string"=w390) -> ("trimmed string"=w389:string)  [unwired: 1 in]
            n148 = Match Pattern(string=w389, regular expression="^[/][/]+") -> (after substring=w391:string)  [unwired: 1 in, 3 out]
            n149 = call <vilib>:"Trim Whitespace.vi"("string"=w391) -> ("trimmed string"=w383:string)  [unwired: 1 in]
            n150 = local write "Comments"(w383) -> ()
            n151 = call <vilib>:"Add State(s) to Queue__JKI_lib_State_Machine.vi"("State(s) in (\"\")"=w384) -> ("States Out"=w385:string)  [unwired: 14 in]
          }
          frame "UI: Cursor Set" {
            # "#CSM \"UI: Cursor Set\"\nSet and Unset Cursor Busy.\n(Usage: \"UI: Cursor Set >> Busy|Idle\")"
            # "Argument"
            n152 = disable-structure shown="Default" {
              disable-tunnel: w399 -> [w405 w410]
              disable-tunnel: [w404 w410] -> w398
              disable-tunnel: w397 -> [w403 _]
              frame condition #0 (active) {
                n153 = case shown="\"Idle\", Default" w403 {
                  tunnel: w405 -> [w407 w409]
                  tunnel: [w406 w408] -> w404
                  frame "Idle", Default {
                    n154 = call <vilib>:"Unset Busy.vi"("error in (no error)"=w407) -> ("error out"=w406:errorcluster)  [unwired: 10 in]
                  }
                  frame "Busy" {
                    n155 = call <vilib>:"Set Busy.vi"("error in (no error)"=w409) -> ("error out"=w408:errorcluster)  [unwired: 9 in, 1 out]
                  }
                }
              }
              frame condition #1 {
              }
            }
            n156 = call <vilib>:"Add State(s) to Queue__JKI_lib_State_Machine.vi"("State(s) in (\"\")"=w402) -> ("States Out"=w401:string)  [unwired: 14 in]
          }
          frame "UI: Front Panel State" {
            # "#CSM \"UI: Front Panel State\"\nSet Front Panel Open or Closed\n(Usage: \"UI: Front Panel State >> Open|Close\")"
            # "Argument"
            n157 = Unbundle By Name(w414) -> ("Core.Current VI Reference"=w413:refnum<vi>)
            n158 = call <vilib>:"Add State(s) to Queue__JKI_lib_State_Machine.vi"("State(s) in (\"\")"=w418) -> ("States Out"=w417:string)  [unwired: 14 in]
            n159 = case shown="\"Close\", \"Closed\"" w412 {
              tunnel: w416 -> [w424 w439 w450 w463 w476]
              tunnel: [w426 w440 w452 w465 w478] -> w415
              tunnel: w413 -> [w425 w437 w451 w464 w477]
              frame "Open", "Standard", Default {
                w419 = T4."Standard" ("State")
                n160 = property class="VI"(reference=w425, error in=w424) -> (reference out=w422:refnum<vi>, error out=w423:errorcluster, "FP.State"=w421:T4)
                n161 = Not Equal?(x=w421, y=w419) -> (x != y?=w420:bool)
                n162 = case shown="True" w420 {
                  tunnel: [w430 w432] -> w426
                  tunnel: w423 -> [w429 w432]
                  tunnel: w422 -> [w428 _]
                  tunnel: w419 -> [w427 _]
                  frame True {
                    n163 = invoke class="VI" method="FP.Open"(reference=w428, error in=w429, "Activate"=TRUE, "State"=w427) -> (error out=w430:errorcluster)  [unwired: 1 in, 4 out]
                  }
                  frame False {
                  }
                }
              }
              frame "Close", "Closed" {
                n164 = property class="VI"(reference=w437, error in=w439) -> (reference out=w436:refnum<vi>, error out=w438:errorcluster, "FP.State"=w434:T4)
                n165 = Not Equal?(x=w434, y=T4."Closed" ("Front Panel Window:State")) -> (x != y?=w433:bool)
                n166 = case shown="False" w433 {
                  tunnel: [w441 w444] -> w440
                  tunnel: w438 -> [w441 w443]
                  tunnel: w436 -> [_ w442]
                  frame False {
                  }
                  frame True {
                    n167 = invoke class="VI" method="FP.Close"(reference=w442, error in=w443) -> (error out=w444:errorcluster)  [unwired: 1 in, 2 out]
                  }
                }
              }
              frame "Hidden", "Hide" {
                w445 = T4."Hidden" ("State")
                n168 = property class="VI"(reference=w451, error in=w450) -> (reference out=w448:refnum<vi>, error out=w449:errorcluster, "FP.State"=w447:T4)
                n169 = Not Equal?(x=w447, y=w445) -> (x != y?=w446:bool)
                n170 = case shown="True" w446 {
                  tunnel: [w456 w457] -> w452
                  tunnel: w449 -> [w455 w457]
                  tunnel: w448 -> [w454 _]
                  tunnel: w445 -> [w453 _]
                  frame True {
                    n171 = invoke class="VI" method="FP.Open"(reference=w454, error in=w455, "State"=w453) -> (error out=w456:errorcluster)  [unwired: 2 in, 4 out]
                  }
                  frame False {
                  }
                }
              }
              frame "Minimize", "Minimized" {
                w458 = T4."Minimized" ("State")
                n172 = property class="VI"(reference=w464, error in=w463) -> (reference out=w461:refnum<vi>, error out=w462:errorcluster, "FP.State"=w460:T4)
                n173 = Not Equal?(x=w460, y=w458) -> (x != y?=w459:bool)
                n174 = case shown="True" w459 {
                  tunnel: [w469 w470] -> w465
                  tunnel: w462 -> [w468 w470]
                  tunnel: w461 -> [w467 _]
                  tunnel: w458 -> [w466 _]
                  frame True {
                    n175 = invoke class="VI" method="FP.Open"(reference=w467, error in=w468, "State"=w466) -> (error out=w469:errorcluster)  [unwired: 2 in, 4 out]
                  }
                  frame False {
                  }
                }
              }
              frame "Maximize", "Maximized" {
                w471 = T4."Maximized" ("State")
                n176 = property class="VI"(reference=w477, error in=w476) -> (reference out=w474:refnum<vi>, error out=w475:errorcluster, "FP.State"=w473:T4)
                n177 = Not Equal?(x=w473, y=w471) -> (x != y?=w472:bool)
                n178 = case shown="True" w472 {
                  tunnel: [w482 w483] -> w478
                  tunnel: w475 -> [w481 w483]
                  tunnel: w474 -> [w480 _]
                  tunnel: w471 -> [w479 _]
                  frame True {
                    n179 = invoke class="VI" method="FP.Open"(reference=w480, error in=w481, "State"=w479) -> (error out=w482:errorcluster)  [unwired: 2 in, 4 out]
                  }
                  frame False {
                  }
                }
              }
            }
          }
          frame "UI: Update CSM States" {
            n180 = Unbundle By Name(w489) -> ("CSM States"=w487:string, "Selection"=w486:cluster{"end":i32, "start":i32})
            n181 = control-ref of="CSM States"() -> (w488:refnum<vi>)
            n182 = property class="Str"(reference=w488, "Value"=w487) -> (reference out=w485:refnum<vi>)  [unwired: 1 in, 1 out]
            n183 = call "_Highlight CSM Scripts(StringControl).vi"("String Ctrl"=w485) -> ("String Ctrl (dup)"=w484:refnum<vi>)  [unwired: 10 in]
            n184 = property class="Str"(reference=w484, "Text.Selection"=w486) -> ()  [unwired: 1 in, 2 out]
          }
          frame "UI: Update Current Range String" {
            n185 = control-ref of="CSM States"() -> (w500:refnum<vi>)
            n186 = property class="Str"(reference=w500) -> ("Value"=w501:string, "Text.Selection"=w499:T14)  [unwired: 1 in, 2 out]
            n187 = Unbundle By Name(w499) -> ("Selection Start"=w498:u32)
            n188 = call "_scriptEditor CSM State Selection.vi"("Pos"=w498, "single-line text"=w501) -> ("Msg Type"=w494:T3, "Selection"=w493:T2, "Selection 2"=w495:cluster{"end":i32, "start":i32})  [unwired: 7 in]
            "Msg Type" <- w494
            "Selection" <- w493
            n189 = Bundle By Name(cluster=w497, "Selection"=w495, "Msg Type"=w494, "Selection"=w493) -> (w496:T9)
          }
          frame "UI: Update CSM Candidates" {
          }
          frame "UI: Update CSM-VI Candidates" {
          }
          frame "UI: Update Candidate" {
            n190 = Unbundle By Name(w521) -> ("Selection.Sel Type"=w520:T1, "Selection.Selction"=w516:string, "Selection.Ref-String"=w513:string)
            n191 = case shown="\"Msg-Module\"" w520 {
              tunnel: [_ string[] ["<register>", "<unregister>"] string[] ["->"] w528 string[] [] string[] [">>"] string[] ["->", "->|", "-@"] w532 _ string[] ["<broadcast>", "<status>", "<interrupt>"] string[] ["//"] string[] []] -> w517
              tunnel: w513 -> [_ _ _ w527 _ _ _ _ _ _ _ _]
              frame "<unknown>", Default {
              }
              frame "Reg-Oper" {
              }
              frame "Reg-Symbol", "Broadcast-Symbol" {
              }
              frame "Msg-State" {
                n192 = call "Read CSM States By CSM.vi"("CSM Name"=w527) -> ("Array"=w528:string[])  [unwired: 9 in, 1 out]
              }
              frame "Msg-Arg" {
              }
              frame "Msg-ArgSymbol", "Broadcast-ArgSymbol" {
              }
              frame "Msg-Symbol" {
              }
              frame "Msg-Module" {
                n193 = call "Read CSMs.vi"() -> ("Array"=w532:string[])  [unwired: 10 in, 1 out]
              }
              frame "Broadcast-Signal" {
              }
              frame "Broadcast-Oper" {
              }
              frame "Comment-Symbol" {
              }
              frame "Comment-Content" {
              }
            }
            n194 = Build Array(w517) -> (w519:string[][])
            n195 = call <vilib>:"Trim Whitespace.vi"("string"=w516) -> ("trimmed string"=w515:string)  [unwired: 1 in]
            n196 = Transpose 2D Array(2D array=w519) -> (transposed array=w518:string[][])
            n197 = Search 1D Array(1D array=w517, element=w515) -> (index of element=w514:i32)  [unwired: 1 in]
            n198 = property on="Candidates" class="MCListbox (strict)"("ItemNames"=w518, "Value"=w514) -> ()  [unwired: 2 in, 2 out]
          }
          frame "---------- Macro ----------" {
            # "#CSM \"Category Seperator\"\nDo not put any code in this frame."
            n199 = call <vilib>:"Add State(s) to Queue__JKI_lib_State_Machine.vi"("State(s) in (\"\")"=w540) -> ("States Out"=w539:string)  [unwired: 14 in]
          }
          frame "Macro: Initialize" {
            # "#CSM \"Macro: Initialize\"\nInitialization Macro (This is called once, when the VI starts)"
            n200 = call <vilib>:"Add State(s) to Queue__JKI_lib_State_Machine.vi"("State(s) in Front (\"\")"="Data: Initialize\nInitialize Core Data\nEvents: Register\nUI: Initialize\n//UI: Front Panel State >> Open\nUI: Init MainTree\nUI: Init States\nUI: Refresh Inputs\nUI: Update CSM States", "State(s) in (\"\")"=w546) -> ("States Out"=w545:string)  [unwired: 13 in]
          }
          frame "Macro: Exit" {
            # "#CSM \"Macro: Exit\"\nExit Macro (This is called once, when the VI exits)"
            n201 = Unbundle By Name(w555) -> ("Core.Close Panel on Exit?"=w554:bool)
            n202 = Select(t="UI: Front Panel State >> Close", s=w554, f="") -> (s? t:f=w551:string)
            n203 = call <vilib>:"Add State(s) to Queue__JKI_lib_State_Machine.vi"("State(s) in Front (\"\")"="//Exit Sub-Modules ", "State(s) in (\"\")"=w551, "State(s) at Back (\"\")"="Data: Cleanup\nEvents: Unregister\nExit") -> ("States Out"=w549:string)  [unwired: 12 in]
            n204 = call <vilib>:"Add State(s) to Queue__JKI_lib_State_Machine.vi"("State(s) in Front (\"\")"=w549, "State(s) in (\"\")"=w558) -> ("States Out"=w557:string)  [unwired: 13 in]
          }
          frame "---------- API ----------" {
            # "#CSM \"Category Seperator\"\nDo not put any code in this frame."
          }
          frame "API: Set Command" {
            # "#CSM API Example\nCopy/Rename this case for your own API"
            n205 = call "CSM - Revert Arguments-Safe String.vi"("Safe Argurment String"=w566) -> ("Origin Argurment String"=w567:string)  [unwired: 8 in]
            n206 = Bundle By Name(cluster=w570, "CSM States"=w567) -> (w568:T9)
            n207 = call <vilib>:"Add State(s) to Queue__JKI_lib_State_Machine.vi"("State(s) in (\"\")"=w564, "State(s) at Back (\"\")"="UI: Refresh Inputs" ("State(s) in Front (\"\")")) -> ("States Out"=w565:string)  [unwired: 13 in]
          }
          frame "---------- Action ----------" {
            # "#CSM \"Category Seperator\"\nDo not put any code in this frame."
            n208 = call <vilib>:"Add State(s) to Queue__JKI_lib_State_Machine.vi"("State(s) in (\"\")"=w576) -> ("States Out"=w575:string)  [unwired: 14 in]
          }
          frame "Action: Change Comments" {
            n209 = local read "Comments"() -> (w580:string)
            n210 = Unbundle By Name(w583) -> ("CSM States"=w582:string)
            n211 = Match Pattern(string=w582, regular expression="//") -> (before substring=w578:string)  [unwired: 1 in, 3 out]
            n212 = call "Build State String with Comments.vi"("Comments"=w580, "State"=w578) -> ("State with Arguments"=w577:string)  [unwired: 6 in]
            n213 = Bundle By Name(cluster=w583, "CSM States"=w577) -> (w579:T9)
          }
          frame "Action: change Symbol" {
            w590 = " " ("regular expression")
            n214 = Unbundle By Name(w603) -> ("CSM States"=w602:string)
            n215 = Match Pattern(string=w602, regular expression="//") -> (before substring=w598:string, after substring=w599:string)  [unwired: 1 in, 2 out]
            n216 = for {
              tunnel: w598 -> [w613]
              tunnel: string[] ["->|", "-@", "->"] ("regular expression") -> [w612] mode=indexing
              tunnel: [w610] -> _ if=w609
              tunnel: [w608] -> w596
              tunnel: [w607] -> w591
              stop <- w609 stop-if-true
              n217 = Match Pattern(string=w613, regular expression=w612) -> (before substring=w608:string, match substring=w610:string, after substring=w607:string, offset past match=w611:i32)  [unwired: 1 in]
              n218 = Greater Or Equal To 0?(x=w611) -> (x >= 0?=w609:bool)
            }
            n219 = call "CSM - Revert Arguments-Safe String.vi"("Safe Argurment String"=w595) -> ("Origin Argurment String"=w594:string)  [unwired: 8 in]
            n220 = call <vilib>:"Trim Whitespace.vi"("string"=w596) -> ("trimmed string"=w593:string)  [unwired: 1 in]
            n221 = call <vilib>:"Trim Whitespace.vi"("string"=w591) -> ("trimmed string"=w592:string)  [unwired: 1 in]
            n222 = call <vilib>:"Trim Whitespace.vi"("string"=w599) -> ("trimmed string"=w587:string)  [unwired: 1 in]
            n223 = Concatenate Strings(w593, w590, w594, w590, w592) -> (w588:string)
            n224 = call "Build State String with Comments.vi"("Comments"=w587, "State"=w588) -> ("State with Arguments"=w589:string)  [unwired: 6 in]
            n225 = Bundle By Name(cluster=w603, "CSM States"=w589) -> (w600:T9)
          }
          frame "Action: Change State" {
            w631 = " " ("regular expression")
            n226 = Unbundle By Name(w638) -> ("CSM States"=w637:string)
            n227 = Match Pattern(string=w637, regular expression="//") -> (before substring=w633:string, after substring=w634:string)  [unwired: 1 in, 2 out]
            n228 = control-ref of="MainTree"() -> (w621:refnum<vi>)
            n229 = control-ref of="CSM-States"() -> (w628:refnum<vi>)
            n230 = for {
              tunnel: w633 -> [w648]
              tunnel: string[] ["->|", "-@", "->"] ("regular expression") -> [w647] mode=indexing
              tunnel: [w645] -> w619 if=w644
              tunnel: [w643] -> w626
              tunnel: [w642] -> _
              stop <- w644 stop-if-true
              n231 = Match Pattern(string=w648, regular expression=w647) -> (before substring=w643:string, match substring=w645:string, after substring=w642:string, offset past match=w646:i32)  [unwired: 1 in]
              n232 = Greater Or Equal To 0?(x=w646) -> (x >= 0?=w644:bool)
            }
            n233 = property class="LstBox (strict)"(reference=w628) -> ("Item Names"=w630:string[], "Value"=w629:i32)  [unwired: 1 in, 2 out]
            n234 = property class="Tree (strict)"(reference=w621) -> ("Value"=w622:string)  [unwired: 1 in, 2 out]
            n235 = Index Array(array=w630, index=w629) -> (element=w625:string)
            n236 = call <vilib>:"Trim Whitespace.vi"("string"=w634) -> ("trimmed string"=w614:string)  [unwired: 1 in]
            n237 = Match Pattern(string=w626, regular expression=">>") -> (after substring=w624:string)  [unwired: 1 in, 3 out]
            n238 = Match Pattern(string=w622, regular expression="/") -> (after substring=w618:string)  [unwired: 1 in, 3 out]
            n239 = call <vilib>:"Trim Whitespace.vi"("string"=w618) -> ("trimmed string"=w617:string)  [unwired: 1 in]
            n240 = call <vilib>:"Build State String with Arguments__JKI_lib_State_Machine.vi"("Arguments (\"\")"=w624, "State"=w625) -> ("State with Arguments"=w623:string)  [unwired: 4 in]
            n241 = Concatenate Strings(w623, w631, w619, w631, w617) -> (w615:string)
            n242 = call "Build State String with Comments.vi"("Comments"=w614, "State"=w615) -> ("State with Arguments"=w616:string)  [unwired: 6 in]
            n243 = Bundle By Name(cluster=w638, "CSM States"=w616) -> (w635:T9)
          }
          frame "Action: clear arguments" {
            w659 = " " ("regular expression")
            n244 = Unbundle By Name(w666) -> ("CSM States"=w665:string)
            n245 = Match Pattern(string=w665, regular expression="//") -> (before substring=w661:string, after substring=w662:string)  [unwired: 1 in, 2 out]
            n246 = for {
              tunnel: w661 -> [w676]
              tunnel: string[] ["->|", "-@", "->"] ("regular expression") -> [w675] mode=indexing
              tunnel: [w673] -> w655 if=w672
              tunnel: [w671] -> w657
              tunnel: [w670] -> w650
              stop <- w672 stop-if-true
              n247 = Match Pattern(string=w676, regular expression=w675) -> (before substring=w671:string, match substring=w673:string, after substring=w670:string, offset past match=w674:i32)  [unwired: 1 in]
              n248 = Greater Or Equal To 0?(x=w674) -> (x >= 0?=w672:bool)
            }
            n249 = call <vilib>:"Trim Whitespace.vi"("string"=w662) -> ("trimmed string"=w652:string)  [unwired: 1 in]
            n250 = Match Pattern(string=w657, regular expression=">>") -> (before substring=w651:string)  [unwired: 1 in, 3 out]
            n251 = call <vilib>:"Trim Whitespace.vi"("string"=w650) -> ("trimmed string"=w649:string)  [unwired: 1 in]
            n252 = call <vilib>:"Build State String with Arguments__JKI_lib_State_Machine.vi"("State"=w651) -> ("State with Arguments"=w656:string)  [unwired: 5 in]
            n253 = Concatenate Strings(w656, w659, w655, w659, w649) -> (w653:string)
            n254 = call "Build State String with Comments.vi"("Comments"=w652, "State"=w653) -> ("State with Arguments"=w654:string)  [unwired: 6 in]
            n255 = Bundle By Name(cluster=w666, "CSM States"=w654) -> (w663:T9)
          }
          frame "Action: Replace Selction" {
            n256 = Unbundle By Name(w692) -> ("Selection.start"=w690:i32, "Selection.end"=w691:i32)
            n257 = property on="CSM States" class="Str"() -> ("Value"=w687:string)  [unwired: 2 in, 2 out]
            n258 = Subtract(x=w691, y=w690) -> (x-y=w689:i32)
            n259 = call "CSM - Revert Arguments-Safe String.vi"("Safe Argurment String"=w688) -> ("Origin Argurment String"=w682:string)  [unwired: 8 in]
            n260 = control-ref of="CSM States"() -> (w685:refnum<vi>)
            n261 = Replace Substring(2:w689, 3:w690, 4:w682, 5:w687) -> (1:w681:string)  [unwired: 1 out]
            n262 = property class="Str"(reference=w685, "Value"=w681) -> (reference out=w679:refnum<vi>)  [unwired: 1 in, 1 out]
            n263 = String Length(string=w681) -> (length=w680:i32)
            n264 = Search/Split String(string=w681, search string/char (-)=w682) -> (substring before match=w683:string, match + rest of string=w684:string, offset of match=w677:i32)  [unwired: 1 in]
            n265 = String Length(string=w682) -> (length=w686:i32)
            n266 = Add(x=w677, y=w686) -> (x+y=w678:i32)
            n267 = call "_Highlight CSM Scripts(StringControl).vi"("String Ctrl"=w679) -> ()  [unwired: 10 in, 1 out]
            n268 = flat-sequence {
              tunnel: w684 -> [_]
              tunnel: w683 -> [_]
              tunnel: w680 -> [_]
              frame #0 {
              }
            }
            n269 = Bundle By Name(cluster=w692, "Selection.start"=w677, "Selection.end"=w678, "CSM States"=w681) -> (w693:T9)
          }
          frame "Action: Move Focus to Edit" {
            n270 = property on="CSM States" class="Str"("Key Focus"=TRUE) -> ()  [unwired: 2 in, 2 out]
          }
          frame "Action: Move to Next Part2" {
            n271 = property on="CSM States" class="Str"() -> ("Value"=w703:string, "Key Focus"=w706:bool, "Text.Selection End"=w705:u32, "Text.Selection Start"=w704:u32)  [unwired: 2 in, 2 out]
            n272 = Max & Min(x=w705, y=w704) -> (min(x,y)=w702:u32)  [unwired: 1 out]
            n273 = case shown="True" w706 {
              tunnel: w703 -> [_ w718]
              tunnel: w702 -> [_ w711]
              frame False {
              }
              frame True {
                n274 = call "_scriptEditor Parse CSM State.vi"("single-line text"=w718) -> ("comments"=w719:T15, "Array"=w717:string[])  [unwired: 8 in, 1 out]
                n275 = Cluster To Array(cluster=w719) -> (array=w716:string[])
                n276 = Build Array (concatenate)(w717, w716) -> (w715:string[])
                n277 = String Length(string=w715) -> (length=w714:i32[])
                n278 = for {
                  tunnel: w714 -> [w723] mode=indexing
                  shift-right: [w720] -> _
                  shift-left: u32 0 -> [w724]
                  tunnel: w711 -> [w722]
                  tunnel: [w720] -> w712
                  stop <- w721 stop-if-true
                  n279 = Add(x=w723, y=w724) -> (x+y=w720:u32)
                  n280 = Greater?(x=w720, y=w722) -> (0:w721:bool)
                }
                n281 = property on="CSM States" class="Str"("Text.Selection End"=w712, "Text.Selection Start"=w712) -> ()  [unwired: 2 in, 2 out]
              }
            }
          }
          frame "Action: Move to Previous Part" {
            n282 = property on="CSM States" class="Str"() -> ("Value"=w726:string, "Key Focus"=w729:bool, "Text.Selection End"=w728:u32, "Text.Selection Start"=w727:u32)  [unwired: 2 in, 2 out]
            n283 = Max & Min(x=w728, y=w727) -> (min(x,y)=w725:u32)  [unwired: 1 out]
            n284 = case shown="True" w729 {
              tunnel: w726 -> [_ w747]
              tunnel: w725 -> [_ w739]
              frame False {
              }
              frame True {
                n285 = call "_scriptEditor Parse CSM State.vi"("single-line text"=w747) -> ("comments"=w748:T15, "Array"=w746:string[])  [unwired: 8 in, 1 out]
                n286 = Cluster To Array(cluster=w748) -> (array=w745:string[])
                n287 = Build Array (concatenate)(w746, w745) -> (w744:string[])
                n288 = String Length(string=w744) -> (length=w743:i32[])
                n289 = for {
                  tunnel: w743 -> [w757] mode=indexing
                  shift-right: [w755] -> _
                  shift-left: u32 0 -> [w756]
                  tunnel: [w756] -> w741 mode=indexing
                  n290 = Add(x=w757, y=w756) -> (x+y=w755:u32)
                }
                n291 = Build Array (concatenate)(u32 0, w741) -> (w734:u32[])
                n292 = for {
                  tunnel: w734 -> [w754] mode=indexing
                  tunnel: w739 -> [w753]
                  shift-right: [w751] -> _
                  shift-left: FALSE -> [w752]
                  tunnel: [w750] -> w737 if=w749
                  i -> [w750]
                  stop <- w749 stop-if-true
                  n293 = Less Or Equal?(x=w754, y=w753) -> (x <= y?=w751:bool)
                  n294 = Less?(x=w751, y=w752) -> (x < y?=w749:bool)
                }
                n295 = Decrement(x=w737) -> (x-1=w736:i32)
                n296 = Index Array(array=w734, index=w736) -> (element=w735:u32)
                n297 = property on="CSM States" class="Str"("Text.Selection End"=w735, "Text.Selection Start"=w735) -> ()  [unwired: 2 in, 2 out]
              }
            }
          }
          frame "Action: Move to Next Part" {
            n298 = property on="CSM States" class="Str"() -> ("Value"=w759:string, "Key Focus"=w762:bool, "Text.Selection End"=w761:u32, "Text.Selection Start"=w760:u32)  [unwired: 2 in, 2 out]
            n299 = Max & Min(x=w761, y=w760) -> (min(x,y)=w758:u32)  [unwired: 1 out]
            n300 = case shown="True" w762 {
              tunnel: w759 -> [_ w779]
              tunnel: w758 -> [_ w771]
              frame False {
              }
              frame True {
                n301 = call "_scriptEditor Parse CSM State.vi"("single-line text"=w779) -> ("comments"=w780:T15, "Array"=w778:string[])  [unwired: 8 in, 1 out]
                n302 = Cluster To Array(cluster=w780) -> (array=w777:string[])
                n303 = Build Array (concatenate)(w778, w777) -> (w776:string[])
                n304 = String Length(string=w776) -> (length=w775:i32[])
                n305 = for {
                  tunnel: w775 -> [w789] mode=indexing
                  shift-right: [w787] -> _
                  shift-left: u32 0 -> [w788]
                  tunnel: [w788] -> w773 mode=indexing
                  n306 = Add(x=w789, y=w788) -> (x+y=w787:u32)
                }
                n307 = Build Array (concatenate)(u32 0, w773) -> (w768:u32[])
                n308 = for {
                  tunnel: w768 -> [w786] mode=indexing
                  tunnel: w771 -> [w785]
                  shift-right: [w783] -> _
                  shift-left: FALSE -> [w784]
                  tunnel: [w782] -> w767 if=w781
                  i -> [w782]
                  stop <- w781 stop-if-true
                  n309 = Less Or Equal?(x=w786, y=w785) -> (x <= y?=w783:bool)
                  n310 = Less?(x=w783, y=w784) -> (x < y?=w781:bool)
                }
                n311 = Index Array(array=w768, index=w767) -> (element=w769:u32)
                n312 = property on="CSM States" class="Str"("Text.Selection End"=w769, "Text.Selection Start"=w769) -> ()  [unwired: 2 in, 2 out]
              }
            }
          }
        }
      }
      n313 = Unbundle By Name(w10) -> ("CSM States"=w9:string)
    }
    frame Error {
    }
  }
  "Error out" <- w4
  "Command out" <- w1
